vi "DAQNavi Read (Counter 2D Pulse Width NChan NSamp).vi"(8 "error in (no error)":errorcluster, 9 "number of samples per channel to read":u32=10, 10 "timeout":dbl=10.0, 11 "task in":i32) -> (0 "error out":errorcluster, 2 "data":cluster{"high period":dbl, "low period":dbl}[][](array[cluster]), 3 "task out":i32)   [LabVIEW 2020]
uses:
  DAQNavi_LV.dll
panel:
  in  "pulse width 2":cluster{"high period":dbl, "low period":dbl}
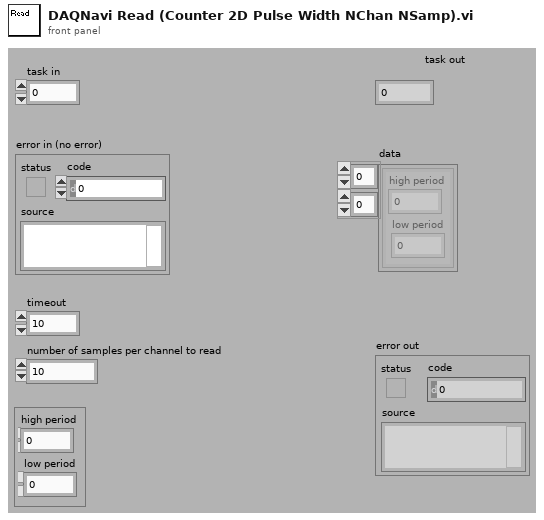
[diagram p1: front panel]
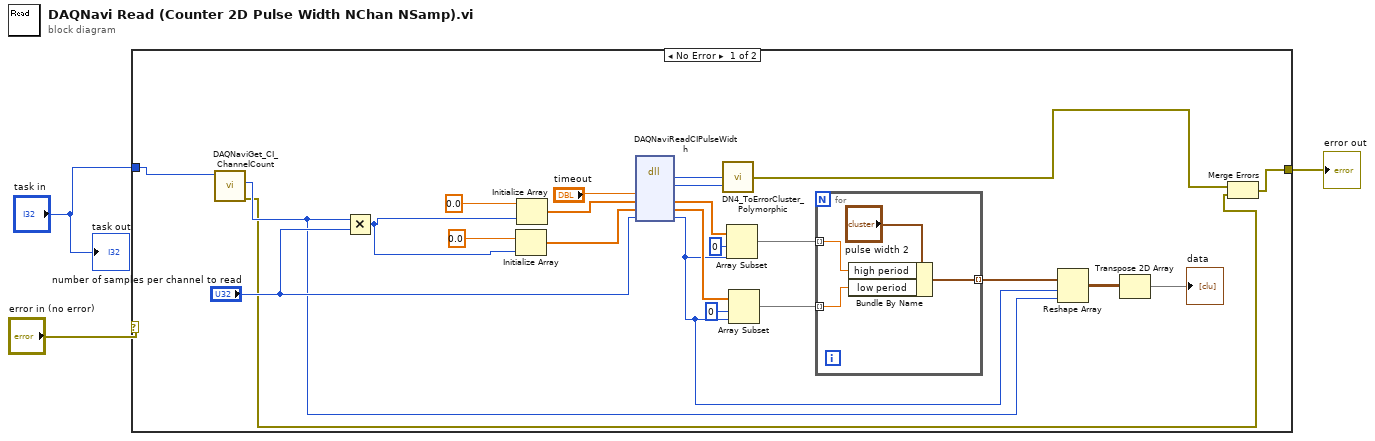
[diagram p0: block diagram]
diagram:
  n1 = case shown="No Error" "error in (no error)" {
    selector: "error in (no error)" -> [_ w32]
    tunnel: [w4 w32] -> w2
    tunnel: "task in" -> [w14 _]
    frame No Error {
      n2 = call "DAQNaviGet_CI_ChannelCount.vi"("task in"=w14) -> ("error out"=w5:errorcluster, "channel count"=w9:i32)  [unwired: 1 in, 8 out]
      n3 = Multiply(x=w9, y="number of samples per channel to read") -> (x*y=w12:u32)
      n4 = Initialize Array(0.0 ("element"), w12) -> (w18:dbl[])
      n5 = Initialize Array(0.0 ("element"), w12) -> (w19:dbl[])
      n6 = dll-call lib="DAQNavi_LV.dll" fn="DAQNaviReadCIPulseWidth"("timeout"="timeout", "hiPeriod"=w19, "loPeriod"=w18, "samples"="number of samples per channel to read") -> ("return type"=w27:i32, "taskID"=w15:i32, "hiPeriod"=w22:dbl[], "loPeriod"=w24:dbl[], "samples"=w10:u32)  [unwired: 4 in, 3 out]
      n7 = call "DN4_ToErrorCluster_Polymorphic.vi"("task id"=w15, "error code"=w27) -> ("error out"=w6:errorcluster)  [unwired: 3 out]
      n8 = Array Subset(array=w22, index=0, length=w10) -> (w17:dbl[])
      n9 = Array Subset(array=w24, index=0, length=w10) -> (w16:dbl[])
      n10 = for {
        tunnel: w17 -> [w31] mode=indexing
        tunnel: w16 -> [w30] mode=indexing
        tunnel: [w29] -> w11 mode=indexing
        n11 = Bundle By Name(cluster="pulse width 2", "high period"=w31, "low period"=w30) -> (w29:cluster{"high period":dbl, "low period":dbl})
      }
      n12 = Reshape Array(w11, w10, w9) -> (w8:cluster{"high period":dbl, "low period":dbl}[][])
      n13 = Transpose 2D Array(2D array=w8) -> (transposed array=→"data":cluster{"high period":dbl, "low period":dbl}[][])
      n14 = Merge Errors(w6, w5) -> (w4:errorcluster)
    }
    frame Error {
    }
  }
  "error out" <- w2
  "task out" <- "task in"
